vi "WinHostToFlexRIO.vi"() -> ()   [LabVIEW 2013]
uses:
  <vilib>/userdefined/High Color/nirio_resource_hc.ctl
  <vilib>/FPGAPlugInAG/PXIe-7966R/niLvFpga_Open_PXIe-7966R.vi
  <vilib>/FPGAPlugInAG/PXIe-7966R/niLvFpga_Reset_PXIe-7966R.vi
  <vilib>/Utility/error.llb/Error Cluster From Error Code.vi
  <vilib>/rvi/errors/niLvFpgaAdjustHostInterfaceError.vi
  <vilib>/FPGAPlugInAG/PXIe-7966R/niLvFpga_Run_PXIe-7966R.vi
  <vilib>/rvi/interface/common/niFpgaWaitOnOcc.vi
  <vilib>/measure/maspectr.llb/FFT Spectrum (Mag-Phase) for 1 Chan.vi
  <vilib>/FPGAPlugInAG/PXIe-7966R/niLvFpga_Close_PXIe-7966R.vi
  <vilib>/rvi/interface/nirviOpenFPGA/nirviOpenFPGA.xnode
  FPGA Bitfiles/FlexRIOMod5761_7966v1_1.lvbitx
  <vilib>/rvi/interface/nirviMethod/nirviMethod.xnode
  <vilib>/rvi/interface/nirviReadWriteControl/nirviReadWriteControl.xnode
  Control 1.ctl
  <vilib>/rvi/interface/nirviCloseFPGA/nirviCloseFPGA.xnode
  <vilib>/measure/NI_MAPro.lvlib
  NiFpgaLv.dll
  <vilib>/rvi/errors/niLvFpgaMergeErrorWithErrorCode.vi
  <vilib>/FPGAPlugInAG/PXIe-7966R/niLvFpga_ReadFifo_PXIe-7966R.vi
  <vilib>/FPGAPlugInAG/PXIe-7966R/niLvFpga_ConfigureFifo_PXIe-7966R.vi
  <vilib>/FPGAPlugInAG/PXIe-7966R/niLvFpga_StartFifo_PXIe-7966R.vi
  <vilib>/FPGAPlugInAG/PXIe-7966R/niLvFpga_StopFifo_PXIe-7966R.vi
panel:
  out "x*y":dbl
  out "DMATtoHOSTOverflows":u16
  out "Elements Remaining":u32
  in  "IgnoreRIOAdapterCorrect":bool
  in  "BlockstoFFT":dbl=1000.0
  in  "Blocktoread":u32=4096
  out "stop 2":bool
  out "Programmed Sampling Rate0":u32
  in  "SGSignalType1":enum16{"DC", "Sine", "Square", "Triangle"}(ring)
  out "Power spectrum graph":cluster{"f0":dbl, "df":dbl, "magnitude":dbl[]}[](graph)
  in  "SGAmp1":u16
  in  "AO1":i32
  in  "SGPhase1":u32
  in  "SGFreq1":u32 format="%.2p"
  in  "SGUpdateRate1":u32
  in  "AOEnable1":bool
  in  "FlexRIO device":T1
  out "DMA0 output":waveform(i16)[](graph)
  in  "SGSignalType0":enum16{"DC", "Sine", "Square", "Triangle"}(ring)
  in  "stop":bool
  out "auxAI9":i16
  out "SGNo":u8
  in  "SGAmp0":u16
  in  "Desired SamplingRate0":u32=10000 format="%.2p"
  in  "DMATtoHOSTEnable0":bool
  in  "AO0":i16
  in  "SGFreq0":u32 format="%.2p"
  in  "SGPhase0":u32
  in  "SGUpdateRate0":u32=10
  in  "AOEnable0":bool
  in  "DebugMode":bool
  in  "DAQStartStop":bool
  out "error out":errorcluster
  out "DMATtoHOSTBlockNWords":u16[](array[numeric])
  out "DMATtoHOSTSampleSize":u8[](array[numeric])
  out "DMATtoHOSTNCh":u16[](array[numeric])
  out "DMATtoHOSTFrameType":u8[](array[numeric])
  out "DevProfile":u8
  out "DevTemp":i16
  out "DevQualityStatus":u8
  out "Fref":u32
  out "RIOAdapterCorrect":bool
  out "Expected IO Module ID":u32
  out "InsertedIOModule ID":u32
  out "FPGAVIversion":u8[](array[numeric])
  out "Platform":enum8{"FlexRIO", "cRIO", "RSeries"}(ring)
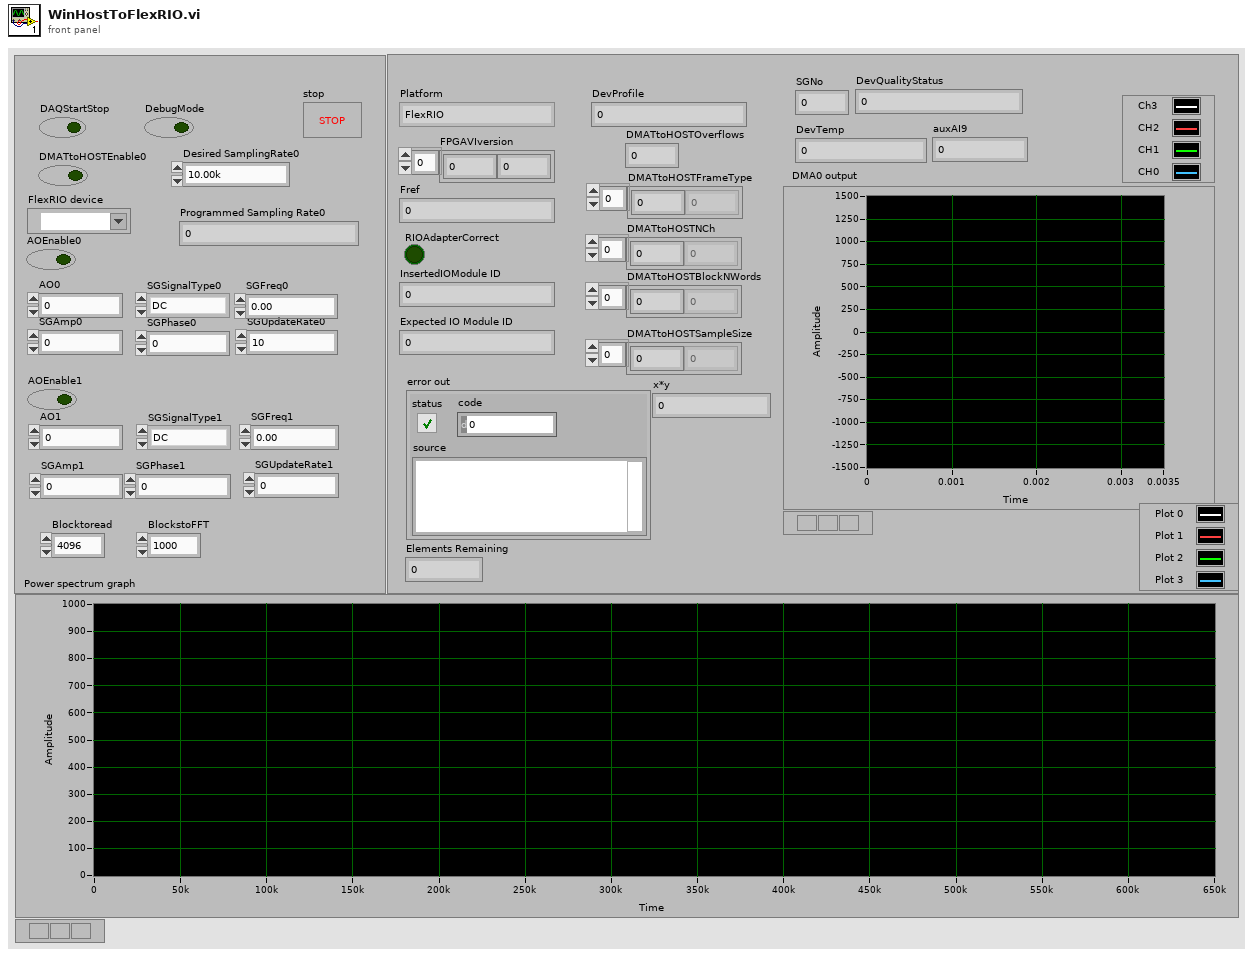
[diagram p1: front panel]
types:
  T1 = typedef "nirio_resource_hc.ctl" = tag
  T2 = enum16{"DAQ-CPU", "IMAQ-CPU", "DAQ-GPU", "IMAQ-GPU"}
  T3 = typedef "Control 1.ctl" = u16
  T4 = cluster{"Timeout":u8, "Timeout":T3, "Timeout":u8, "Timeout":u16}
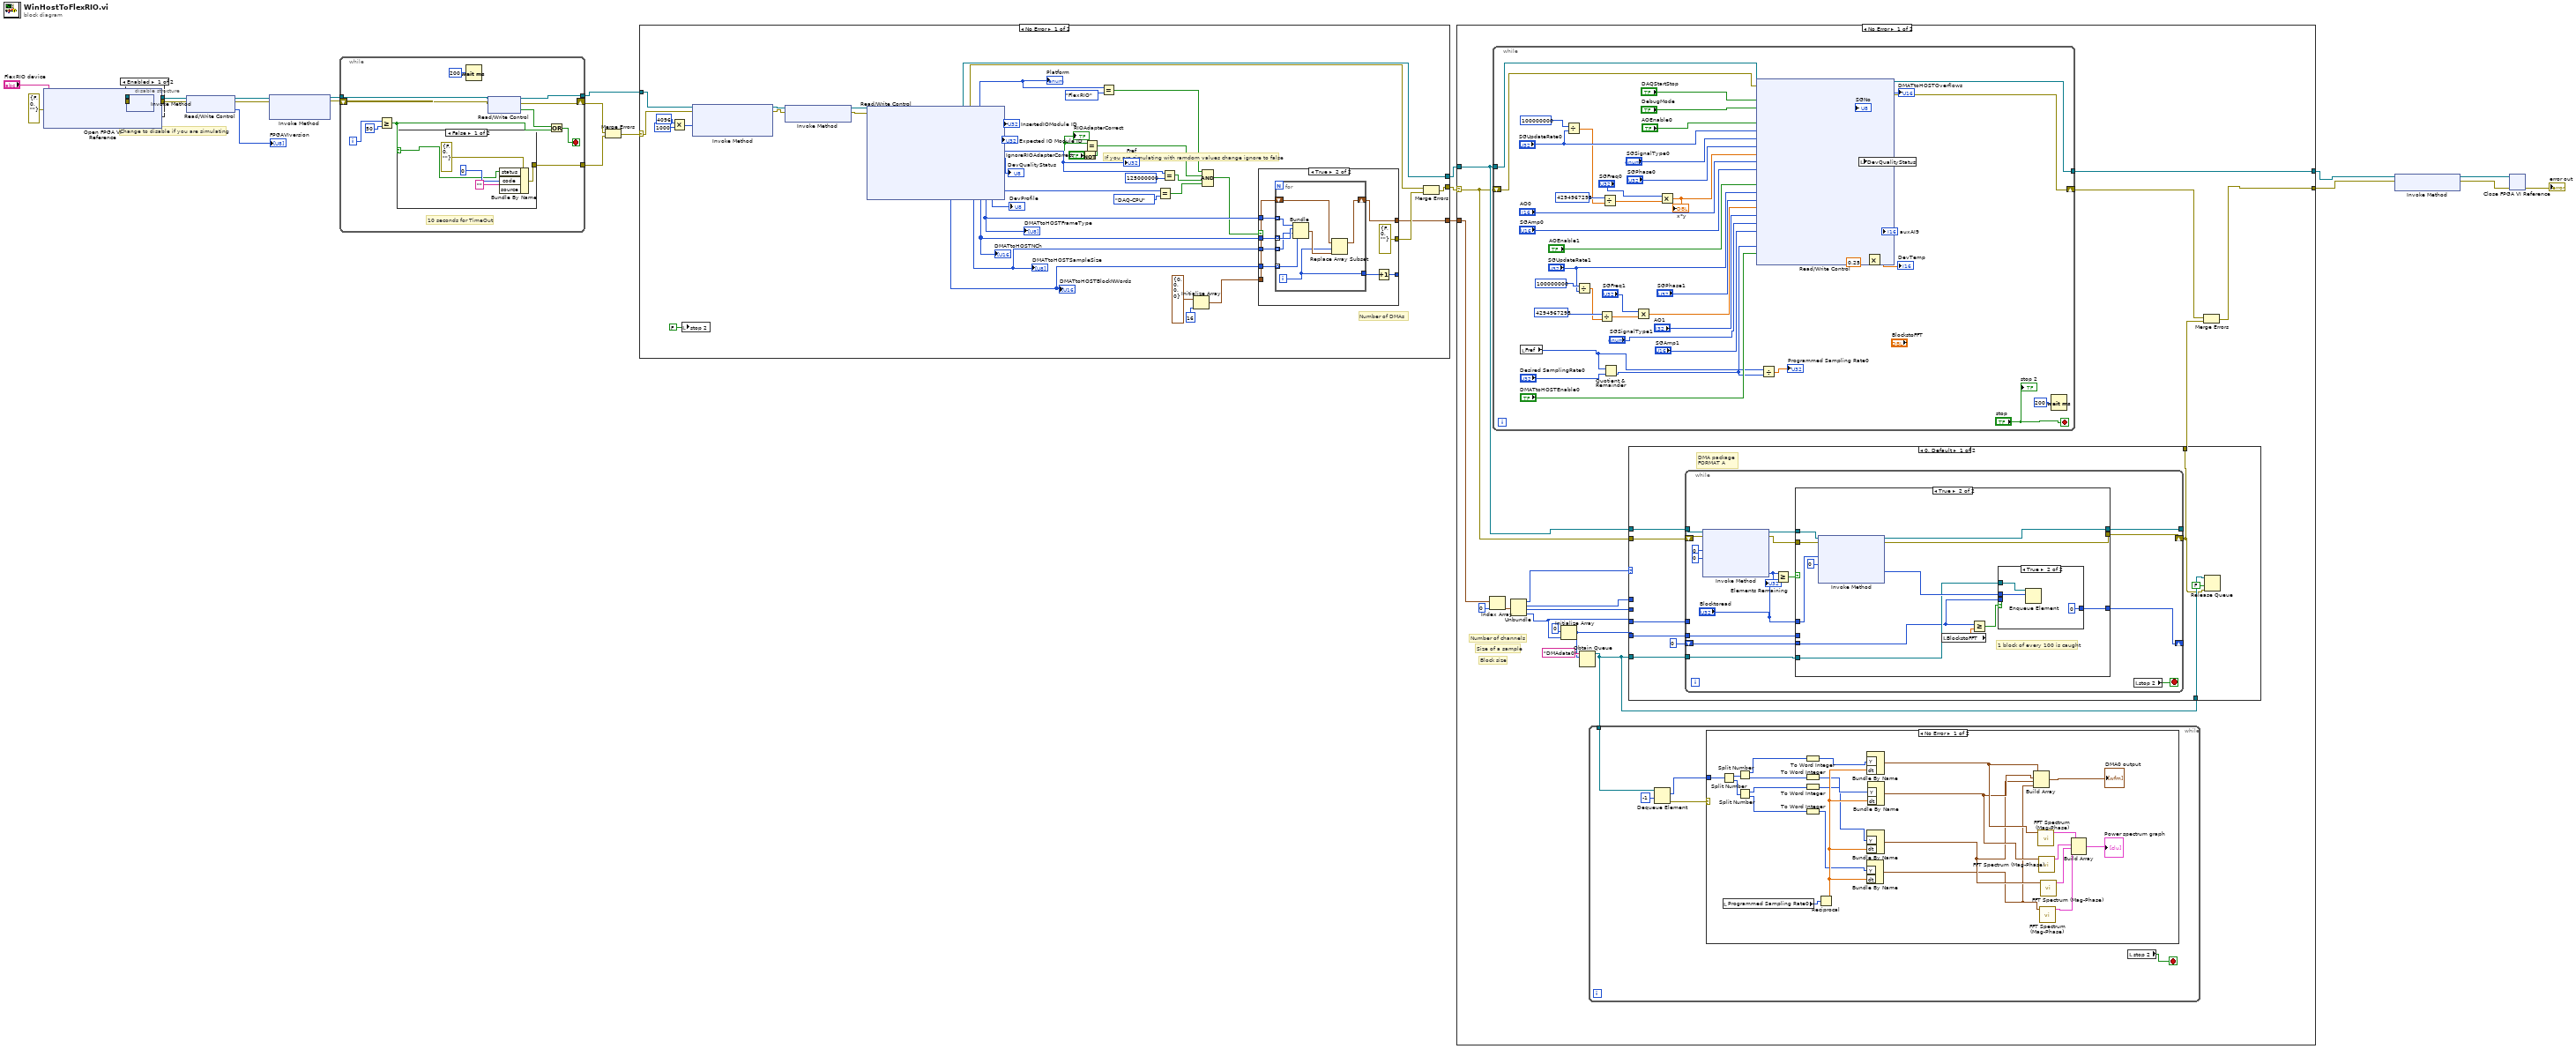
[diagram p0: block diagram]
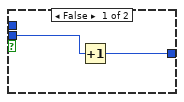
[diagram p5: hidden frame]
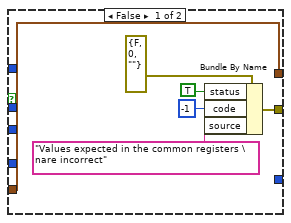
[diagram p8: hidden frame]
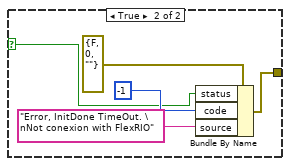
[diagram p10: hidden frame]
diagram:
  # "Change to disable if you are simulating"
  n1 = xnode "Open FPGA VI Reference"("error in"=errorcluster {"status"=FALSE, "code"=0, "source"=""}, "resource name"="FlexRIO device") -> ("FPGA VI Reference Out"=w22:refnum<k20>, "error out"=w23:errorcluster)
  n2 = disable-structure shown="Enabled" {
    disable-tunnel: w23 -> [w27 w28]
    disable-tunnel: w22 -> [w26 w29]
    disable-tunnel: [w25 w29] -> w9
    disable-tunnel: [w24 w28] -> w8
    frame Enabled {
      n3 = xnode "Invoke Method"("FPGA VI Reference In"=w26, "error in"=w27) -> ("FPGA VI Reference Out"=w25:refnum<k20>, "error out"=w24:errorcluster)
    }
    frame Disabled {
    }
  }
  n4 = xnode "Read/Write Control"("FPGA VI Reference In"=w9, "error in"=w8) -> ("FPGA VI Reference Out"=w7:refnum<k20>, "error out"=w6:errorcluster, "FPGAVIversion"=→"FPGAVIversion":u8[])
  n5 = xnode "Invoke Method"("FPGA VI Reference In"=w7, "error in"=w6) -> ("FPGA VI Reference Out"=w20:refnum<k20>, "error out"=w19:errorcluster)  [unwired: 1 in]
  n6 = while {
    tunnel: w20 -> [w40]
    tunnel: [w37] -> w18
    shift-right: [w38] -> w16
    shift-left: w19 -> [w39]
    tunnel: [w30] -> w17
    i -> [w35]
    stop <- w32 stop-if-true
    # "10 seconds for TimeOut"
    n7 = Greater Or Equal?(x=w35, y=50) -> (x >= y?=w31:bool)
    n8 = case shown="False" w31 {
      selector: w31 -> [w42 w47]
      tunnel: [w41 w46] -> w30
      frame False {
        n9 = Bundle By Name(cluster=errorcluster {"status"=FALSE, "code"=0, "source"=""} ("error constant"), "status"=w42, "code"=0, "source"="") -> (w41:errorcluster)
      }
      frame True {
        n10 = Bundle By Name(cluster=errorcluster {"status"=FALSE, "code"=0, "source"=""} ("error constant"), "status"=w47, "code"=-1, "source"="Error, InitDone TimeOut. \nNot conexion with FlexRIO") -> (w46:errorcluster)
      }
    }
    n11 = Wait (ms)(milliseconds to wait=u32 200) -> ()  [unwired: 1 out]
    n12 = xnode "Read/Write Control"("FPGA VI Reference In"=w40, "error in"=w39) -> ("FPGA VI Reference Out"=w37:refnum<k20>, "error out"=w38:errorcluster, "InitDone"=w33:bool)
    n13 = Or(x=w33, y=w31) -> (x .or. y?=w32:bool)
  }
  n14 = Merge Errors(w16, w17) -> (w15:errorcluster)
  n15 = case shown="No Error" w15 {
    selector: w15 -> [w83 w114]
    tunnel: w18 -> [w84 w113]
    tunnel: [w79 w113] -> w12
    tunnel: [w56 w114] -> w13
    tunnel: [w54 _] -> w11
    frame No Error {
      # "If you are simulating with ramdom values change ignore to false"
      # "Number of DMAs"
      n16 = Multiply(x=u32 4096 ("Requested Depth"), y=u32 1000) -> (x*y=w85:u32)
      n17 = local write "stop 2"(FALSE ("stop 2")) -> ()
      n18 = xnode "Invoke Method"("FPGA VI Reference In"=w84, "error in"=w83, "Requested Depth"=w85) -> ("FPGA VI Reference Out"=w89:refnum<k20>, "error out"=w88:errorcluster)  [unwired: 1 out]
      n19 = xnode "Invoke Method"("FPGA VI Reference In"=w89, "error in"=w88) -> ("FPGA VI Reference Out"=w81:refnum<k20>, "error out"=w82:errorcluster)
      n20 = xnode "Read/Write Control"("FPGA VI Reference In"=w81, "error in"=w82) -> ("FPGA VI Reference Out"=w79:refnum<k20>, "error out"=w57:errorcluster, "Platform"=w78:enum8{"FlexRIO", "cRIO", "RSeries"}, "InsertedIOModule ID"=→"InsertedIOModule ID":u32, "Expected IO Module ID"=→"Expected IO Module ID":u32, "RIOAdapterCorrect"=w74:bool, "Fref"=w76:u32, "DevQualityStatus"=→"DevQualityStatus":u8, "DevProfile"=w70:u8, "DMATtoHOSTFrameType"=w65:u8[], "DMATtoHOSTNCh"=w68:T3[], "DMATtoHOSTSampleSize"=w67:u8[], "DMATtoHOSTBlockNWords"=w66:u16[])
      "Platform" <- w78
      "RIOAdapterCorrect" <- w74
      "Fref" <- w76
      "DevProfile" <- w70
      "DMATtoHOSTFrameType" <- w65
      "DMATtoHOSTNCh" <- w68
      "DMATtoHOSTSampleSize" <- w67
      "DMATtoHOSTBlockNWords" <- w66
      n21 = Not(x="IgnoreRIOAdapterCorrect") -> (.not. x?=w51:bool)
      n22 = Equal?(x=w74, y=w51) -> (x = y?=w63:bool)
      n23 = Equal?(x=w78, y=enum16{"FlexRIO", "cRIO", "R-Series"}."FlexRIO") -> (x = y?=w53:bool)
      n24 = Equal?(x=w70, y=T2."DAQ-CPU") -> (x = y?=w61:bool)
      n25 = Equal?(x=w76, y=u32 125000000) -> (x = y?=w62:bool)
      n26 = Initialize Array(cluster{u8, u16, u8, u16} {0, 0, 0, 0}, 16 ("dimension size")) -> (w58:cluster{u8, u16, u8, u16}[])
      n27 = Compound Arithmetic op=AND(w53, w63, w62, w61) -> (w64:bool)
      n28 = case shown="True" w64 {
        tunnel: w68 -> [_ w104]
        tunnel: w67 -> [_ w103]
        tunnel: w66 -> [_ w102]
        tunnel: w65 -> [_ w101]
        tunnel: w58 -> [w90 w100]
        tunnel: [w90 w99] -> w54
        tunnel: [w91 errorcluster {"status"=FALSE, "code"=0, "source"=""} ("error constant")] -> w55
        tunnel: [_ w96] -> _
        frame False {
          n29 = Bundle By Name(cluster=errorcluster {"status"=FALSE, "code"=0, "source"=""} ("error constant"), "status"=TRUE, "code"=-1, "source"="Values expected in the common registers \nare incorrect") -> (w91:errorcluster)
        }
        frame True {
          n30 = for {
            tunnel: w104 -> [w110] mode=indexing
            tunnel: w103 -> [w109] mode=indexing
            tunnel: w102 -> [w108] mode=indexing
            tunnel: w101 -> [w111] mode=indexing
            shift-right: [w106] -> w99
            shift-left: w100 -> [w112]
            tunnel: [w105] -> w97
            i -> [w105]
            n31 = Bundle("Timeout"=w111, "Timeout"=w110, "Timeout"=w109, "Timeout"=w108) -> (w107:T4)  [unwired: 1 in]
            n32 = Replace Array Subset(array=w112, new element=w107, index=w105) -> (w106:cluster{u8, u16, u8, u16}[])
          }
          n33 = Increment(x=w97) -> (x+1=w96:i32)
        }
      }
      n34 = Merge Errors(w57, w55) -> (w56:errorcluster)
    }
    frame Error {
    }
  }
  n35 = case shown="No Error" w13 {
    selector: w13 -> [w124 w251]
    tunnel: w12 -> [w125 w250]
    tunnel: [w131 w250] -> w4
    tunnel: [w116 w251] -> w3
    tunnel: w11 -> [w130 _]
    frame No Error {
      # "Block size"
      # "Size of a sample"
      # "Number of channels"
      n36 = Index Array(array=w130, index=0) -> (element=w128:cluster{u8, u16, u8, u16})
      n37 = while {
        shift-right: [w238] -> w118
        shift-left: w124 -> [w248]
        tunnel: w125 -> [w249]
        tunnel: [w247] -> w131
        stop <- "stop" stop-if-true
        n38 = local read "Fref"() -> (w210:u32)
        n39 = Divide(x=100000000, y="SGUpdateRate0") -> (x/y=w228:dbl)
        n40 = Divide(x=100000000, y="SGUpdateRate1") -> (x/y=w220:dbl)
        n41 = Divide(x=i64 4294967295, y=w220) -> (x/y=w222:dbl)
        n42 = Divide(x=i64 4294967295, y=w228) -> (x/y=w232:dbl)
        n43 = Quotient & Remainder(x=w210, y="Desired SamplingRate0") -> (floor(x/y)=w209:u32)  [unwired: 1 out]
        n44 = Multiply(x="SGFreq1", y=w222) -> (x*y=w218:dbl)
        n45 = Multiply(x="SGFreq0", y=w232) -> (x*y=w230:dbl)
        "x*y" <- w230
        n46 = xnode "Read/Write Control"("FPGA VI Reference In"=w249, "error in"=w248, "DAQStartStop"="DAQStartStop", "DebugMode"="DebugMode", "AOEnable0"="AOEnable0", "SGUpdateRate0"="SGUpdateRate0", "SGSignalType0"="SGSignalType0", "SGPhase0"="SGPhase0", "SGFreq0"=w230, "AO0"="AO0", "SGAmp0"="SGAmp0", "AOEnable1"="AOEnable1", "SGUpdateRate1"="SGUpdateRate1", "SGPhase1"="SGPhase1", "SGFreq1"=w218, "AO1"="AO1", "SGSignalType1"="SGSignalType1", "SGAmp1"="SGAmp1", "DMATtoHOSTSamplingRate0"=w209, "DMATtoHOSTEnable0"="DMATtoHOSTEnable0") -> ("FPGA VI Reference Out"=w247:refnum<k20>, "error out"=w238:errorcluster, "DMATtoHOSTOverflows"=→"DMATtoHOSTOverflows":u16, "SGNo"=→"SGNo":u8, "DevQualityStatus"=w240:u8, "auxAI9"=→"auxAI9":i32, "DevTemp"=w213:i16)
        n47 = Divide(x=w210, y=w209) -> (x/y=→"Programmed Sampling Rate0":dbl)
        n48 = local write "DevQualityStatus"(w240) -> ()
        n49 = Multiply(x=w213, y=sgl 0.25) -> (x*y=→"DevTemp":sgl)
        n50 = Wait (ms)(milliseconds to wait=u32 200) -> ()  [unwired: 1 out]
        "stop 2" <- "stop"
      }
      n51 = Unbundle(w128) -> (w127:u8, w126:u16, w123:u8, w121:u16)
      n52 = Initialize Array(u64 0, w121) -> (w119:u64[])
      n53 = Obtain Queue(name (unnamed)="DMAdata0", element data type=w119) -> (queue out=w115:refnum<queue>)  [unwired: 3 in, 2 out]
      n54 = while {
        tunnel: w115 -> [w133]
        stop <- w135 stop-if-true
        n55 = Dequeue Element(queue=w133, timeout in ms (-1)=-1) -> (element=w136:u64[], error out=w132:errorcluster)  [unwired: 1 in, 2 out]
        n56 = case shown="No Error" w132 {
          tunnel: w136 -> [w159 _]
          frame No Error {
            n57 = Split Number(x=w159) -> (hi(x)=w158:u32[], lo(x)=w157:u32[])
            n58 = local read "Programmed Sampling Rate0"() -> (w152:u32)
            n59 = Split Number(x=w158) -> (hi(x)=w153:u16[], lo(x)=w154:u16[])
            n60 = Split Number(x=w157) -> (hi(x)=w155:u16[], lo(x)=w156:u16[])
            n61 = To Word Integer(number=w153) -> (16bit integer=w145:i16[])
            n62 = To Word Integer(number=w154) -> (16bit integer=w144:i16[])
            n63 = To Word Integer(number=w155) -> (16bit integer=w141:i16[])
            n64 = To Word Integer(number=w156) -> (16bit integer=w140:i16[])
            n65 = Reciprocal(x=w152) -> (1/x=w151:dbl)
            n66 = Bundle By Name("Y"=w140, "dt"=w151) -> (w137:waveform(i16))  [unwired: 1 in]
            n67 = Bundle By Name("Y"=w145, "dt"=w151) -> (w142:waveform(i16))  [unwired: 1 in]
            n68 = Bundle By Name("Y"=w141, "dt"=w151) -> (w138:waveform(i16))  [unwired: 1 in]
            n69 = Bundle By Name("Y"=w144, "dt"=w151) -> (w139:waveform(i16))  [unwired: 1 in]
            n70 = Build Array(w142, w139, w138, w137) -> (→"DMA0 output":waveform(i16)[])
            n71 = call-poly <vilib>:"FFT Spectrum (Mag-Phase).vi"("time signal"=w142) -> ("magnitude"=w150:cluster{"f0":dbl, "df":dbl, "magnitude":dbl[]})  [unwired: 6 in, 4 out]
            n72 = call-poly <vilib>:"FFT Spectrum (Mag-Phase).vi"("time signal"=w139) -> ("magnitude"=w149:cluster{"f0":dbl, "df":dbl, "magnitude":dbl[]})  [unwired: 6 in, 4 out]
            n73 = call-poly <vilib>:"FFT Spectrum (Mag-Phase).vi"("time signal"=w137) -> ("magnitude"=w147:cluster{"f0":dbl, "df":dbl, "magnitude":dbl[]})  [unwired: 6 in, 4 out]
            n74 = call-poly <vilib>:"FFT Spectrum (Mag-Phase).vi"("time signal"=w138) -> ("magnitude"=w148:cluster{"f0":dbl, "df":dbl, "magnitude":dbl[]})  [unwired: 6 in, 4 out]
            n75 = Build Array(w150, w149, w148, w147) -> (→"Power spectrum graph":cluster{"f0":dbl, "df":dbl, "magnitude":dbl[]}[])
          }
          frame Error {
          }
        }
        n76 = local read "stop 2"() -> (w135:bool)
      }
      n77 = case shown="0, Default" w127 {
        tunnel: w126 -> [_ _]
        tunnel: w123 -> [_ _]
        tunnel: w121 -> [w165 _]
        tunnel: w125 -> [w168 _]
        tunnel: w124 -> [w166 w205]
        tunnel: w119 -> [w167 _]
        tunnel: [w160 w205] -> w117
        tunnel: w115 -> [w164 _]
        tunnel: w115 -> [w162 _]
        frame 0, Default {
          # "DMA package \nFORMAT A"
          n78 = while {
            tunnel: w168 -> [w181]
            tunnel: w167 -> [w175]
            tunnel: w165 -> [_]
            tunnel: [w183] -> _
            shift-right: [w182] -> w160
            shift-left: w166 -> [w180]
            tunnel: w164 -> [w172]
            shift-right: [w170] -> _
            shift-left: 0 -> [w171]
            stop <- w184 stop-if-true
            n79 = xnode "Invoke Method"("FPGA VI Reference In"=w181, "error in"=w180, "Number of Elements"=u32 0, "Timeout (ms)"=0) -> ("FPGA VI Reference Out"=w174:refnum<k20>, "error out"=w173:errorcluster, "Elements Remaining"=w177:u32)  [unwired: 1 out]
            "Elements Remaining" <- w177
            n80 = Greater Or Equal?(x=w177, y="Blocktoread") -> (x >= y?=w176:bool)
            n81 = case shown="True" w176 {
              tunnel: [w187 w199] -> w183
              tunnel: [w186 w198] -> w182
              tunnel: "Blocktoread" -> [_ w197]
              tunnel: w175 -> [_ _]
              tunnel: w174 -> [w187 w194]
              tunnel: w173 -> [w186 w193]
              tunnel: w172 -> [_ w192]
              tunnel: w171 -> [w185 w189]
              tunnel: [w185 w188] -> w170
              frame False {
              }
              frame True {
                # "1 block of every 100 is caught"
                n82 = xnode "Invoke Method"("FPGA VI Reference In"=w194, "error in"=w193, "Number of Elements"=w197, "Timeout (ms)"=0) -> ("FPGA VI Reference Out"=w199:refnum<k20>, "error out"=w198:errorcluster, "Data"=w195:u64[])  [unwired: 1 out]
                n83 = local read "BlockstoFFT"() -> (w191:dbl)
                n84 = Greater Or Equal?(x=w189, y=w191) -> (x >= y?=w190:bool)
                n85 = case shown="True" w190 {
                  tunnel: w195 -> [_ w204]
                  tunnel: w192 -> [_ w203]
                  tunnel: w189 -> [w201 _]
                  tunnel: [w200 0] -> w188
                  frame False {
                    n86 = Increment(x=w201) -> (x+1=w200:i32)
                  }
                  frame True {
                    n87 = Enqueue Element(queue=w203, element=w204) -> ()  [unwired: 2 in, 3 out]
                  }
                }
              }
            }
            n88 = local read "stop 2"() -> (w184:bool)
          }
          n89 = Release Queue(queue=w162, force destroy? (F)=FALSE, error in (no error)=w160) -> ()  [unwired: 3 out]
        }
        frame 1 {
        }
      }
      n90 = Merge Errors(w118, w117) -> (w116:errorcluster)
    }
    frame Error {
    }
  }
  n91 = xnode "Invoke Method"("FPGA VI Reference In"=w4, "error in"=w3) -> ("FPGA VI Reference Out"=w2:refnum<k20>, "error out"=w1:errorcluster)
  n92 = xnode "Close FPGA VI Reference"("FPGA VI Reference In"=w2, "error in"=w1) -> ("error out"=→"error out":errorcluster)
